vi "FA_ApplyFIRSTdata.vi"(8 "Error In":errorcluster) -> (0 "Error Out":errorcluster)   [LabVIEW 2014, in "FA_FIRST.lvlib"]
uses:
  FA_FIRST.lvlib
  FA_LocalStore API/source/VI Source/FA_LocalStore.lvlib
  FA_LocalStore API/source/VI Source/FA_LSSpecialTypes.ctl
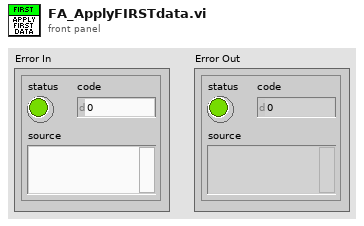
[diagram p1: front panel]
types:
  T1 = typedef "FA_LocalStore.lvlib/FA_LSSpecialTypes.ctl" = string
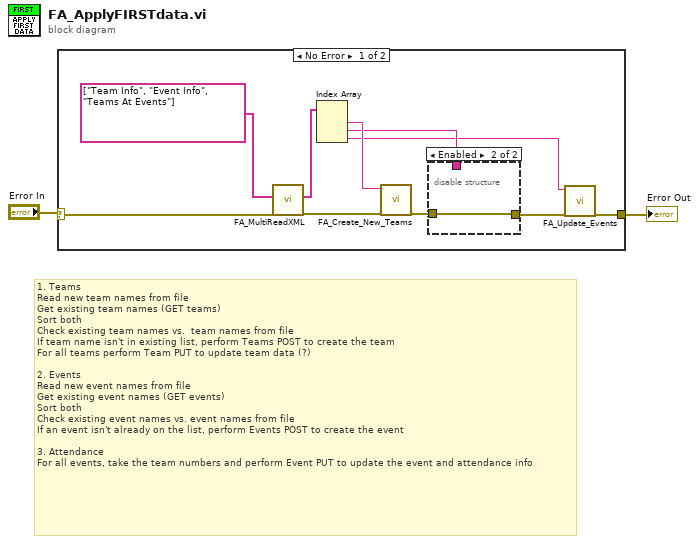
[diagram p0: block diagram]
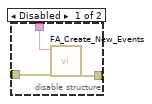
[diagram p2: hidden frame]
diagram:
  # "1. Teams\nRead new team names from file\nGet existing team names (GET teams)\nSort both\nCheck existing team names vs.  team names from file\nIf team name isn't in existing list, perform Teams POST to create the team\nFor all teams perform Team PUT to update team data (?)\n\n2. Events\nRead new event names from file\nGet existing event names (GET events)\nSort both\nCheck existing event names vs. event names from file\nIf an event isn't already on the list, perform Events POST to create the event\n\n3. Attendance\nFor all events, take the team numbers and perform Event PUT to update the event and attendance info"
  n1 = case shown="No Error" "Error In" {
    selector: "Error In" -> [w11 w17]
    tunnel: [w4 w17] -> w1
    frame No Error {
      n2 = call "FA_MultiReadXML.vi"("Error In"=w11, "Special Type Array"=T1[] ["Team Info", "Event Info", "Teams At Events"]) -> ("Error Out"=w8:errorcluster, "XML String Array"=w12:string[])  [unwired: 6 in]
      n3 = Index Array(array=w12) -> (element #1=w9:string, element #2=w5:string, element #3=w3:string)  [unwired: 3 in]
      n4 = call "FA_Create_New_Teams.vi"("error in (no error)"=w8, "XML String"=w9) -> ("error out"=w7:errorcluster)  [unwired: 9 in]
      n5 = disable-structure shown="Enabled" {
        disable-tunnel: w7 -> [w15 w16]
        disable-tunnel: [w14 w16] -> w6
        disable-tunnel: w5 -> [w13 _]
        frame Disabled {
          n6 = call "FA_Create_New_Events.vi"("error in"=w15, "XML String"=w13) -> ("error out"=w14:errorcluster)  [unwired: 9 in]
        }
        frame Enabled {
        }
      }
      n7 = call "FA_Update_Events.vi"("error in (no error)"=w6, "Attendance XML"=w3) -> ("error out"=w4:errorcluster)  [unwired: 9 in]
    }
    frame Error {
    }
  }
  "Error Out" <- w1
